vi "KeyPress.vi"(9 "Millis":u32, 11 "Virtual Key":u8(ring)=65) -> ()   [LabVIEW 2023]
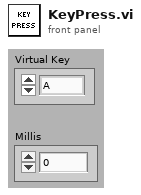
[diagram p1: front panel]
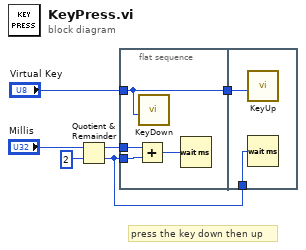
[diagram p0: block diagram]
diagram:
  # "press the key down then up"
  n1 = Quotient & Remainder(x="Millis", y=u32 2) -> (x-y*floor(x/y)=w2:u32, floor(x/y)=w1:u32)
  n2 = flat-sequence {
    tunnel: "Virtual Key" -> [w10]
    tunnel: [w10] -> w5
    tunnel: w2 -> [w9]
    tunnel: w1 -> [w8]
    tunnel: w5 -> [w12]
    tunnel: w1 -> [w11]
    frame #0 {
      n3 = Add(x=w9, y=w8) -> (x+y=w7:u32)
      n4 = call "KeyDown.vi"("Virtual Key"=w10) -> ()  [unwired: 11 in]
      n5 = Wait (ms)(milliseconds to wait=w7) -> ()  [unwired: 1 out]
    }
    frame #1 {
      n6 = call "KeyUp.vi"("Virtual Key"=w12) -> ()  [unwired: 11 in]
      n7 = Wait (ms)(milliseconds to wait=w11) -> ()  [unwired: 1 out]
    }
  }
